vi "Stop Chassis.vi"(8 "error in (no error)":errorcluster, 10 "final error code":i32, 11 "Master Slave in":refnum<class "Master Slave.lvclass">) -> (0 "error out":errorcluster, 2 "Max Read Time (ms)":i32, 3 "Master Slave out":refnum<class "Master Slave.lvclass">)   [LabVIEW 2012, in "Data Acquisition.lvlib" / "Master Slave.lvclass"]
uses:
  Master Slave.lvclass
  Class Chassis Tasks/Chassis Tasks.lvclass/Chassis Tasks.ctl
  <vilib>/ActorFramework/Stop Msg/Stop Msg.lvclass/Stop Msg.ctl
  <vilib>/ActorFramework/Message Enqueuer/Message Enqueuer.lvclass/Message Enqueuer.ctl
  Class Chassis Tasks/Read HS DAQ Task.vi
  Class Chassis Tasks/Read LS DAQ Task.vi
  Class Chassis Tasks/Read LS ActorQ.vi
  <vilib>/ActorFramework/Stop Msg/Send Emergency Stop.vi
  <vilib>/ActorFramework/Stop Msg/Send Normal Stop.vi
  <vilib>/ActorFramework/Message Enqueuer/Enqueue Critical.vi
  <vilib>/ActorFramework/Message Enqueuer/Enqueue.vi
  <vilib>/ActorFramework/Message Priority Queue/Priority Enqueue.vi
  Class DAQ Task/DAQ Task.lvclass
  <vilib>/ActorFramework/Message Enqueuer/Message Enqueuer.lvclass
  <vilib>/ActorFramework/Stop Msg/Stop Msg.lvclass
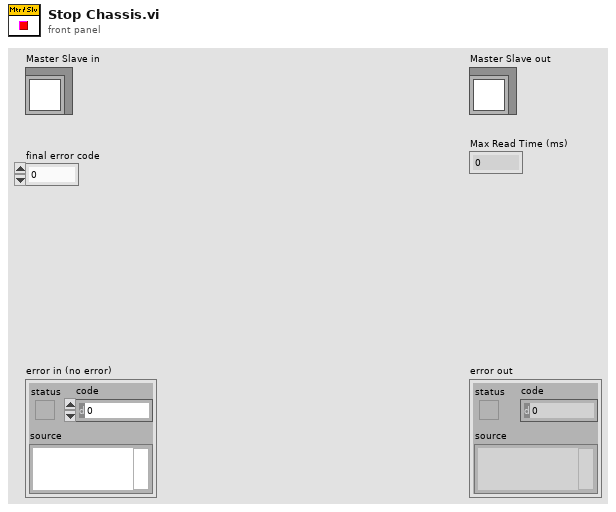
[diagram p1: front panel]
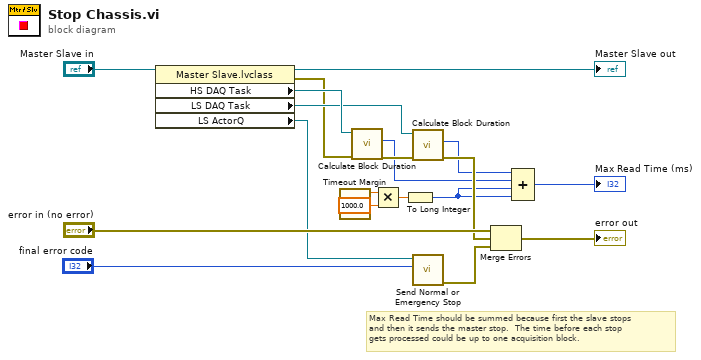
[diagram p0: block diagram]
diagram:
  # "Max Read Time should be summed because first the slave stops\nand then it sends the master stop.  The time before each stop\ngets processed could be up to one acquisition block."
  n1 = property class="Master Slave.lvclass"(reference="Master Slave in") -> (reference out=→"Master Slave out":refnum<class "Master Slave.lvclass">, error out=w8:errorcluster, "HS DAQ Task"=w12:refnum<class "DAQ Task.lvclass">, "LS DAQ Task"=w11:refnum<class "DAQ Task.lvclass">, "LS ActorQ"=w13:refnum<class "Message Enqueuer.lvclass">)  [unwired: 1 in]
  n2 = call "Timeout Margin.vi"() -> ("y"=w4:dbl)  [unwired: 11 in]
  n3 = call "Calculate Block Duration.vi"("error in (no error)"=w8, "DAQ Task in"=w12) -> ("error out"=w9:errorcluster, "Block Duration (ms)"=w6:i32)  [unwired: 7 in, 1 out]
  n4 = Multiply(x=w4, y=1000.0) -> (x*y=w2:dbl)
  n5 = To Long Integer(number=w2) -> (32bit integer=w1:i32)
  n6 = call "Calculate Block Duration.vi"("error in (no error)"=w9, "DAQ Task in"=w11) -> ("error out"=w10:errorcluster, "Block Duration (ms)"=w7:i32)  [unwired: 7 in, 1 out]
  n7 = call <vilib>:"Send Normal or Emergency Stop.vi"("final error code"="final error code", "Message Enqueuer"=w13) -> ("error out"=w17:errorcluster)  [unwired: 9 in]
  n8 = Merge Errors("error in (no error)", w10, w17) -> (→"error out":errorcluster)
  n9 = Compound Arithmetic op=ADD(w7, w6, w1, w1) -> (→"Max Read Time (ms)":i32)
